vi "Add autonmous program.vi"(10 "Programs in":string[](array[string]), 11 "Program Name in":string[](array[string])) -> (2 "Programs out":string[](array[string]), 3 "Program Name out":string[](array[string]))   [LabVIEW 2013]
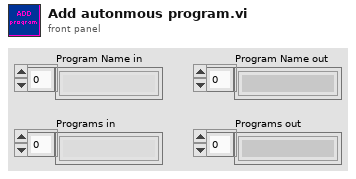
[diagram p1: front panel]
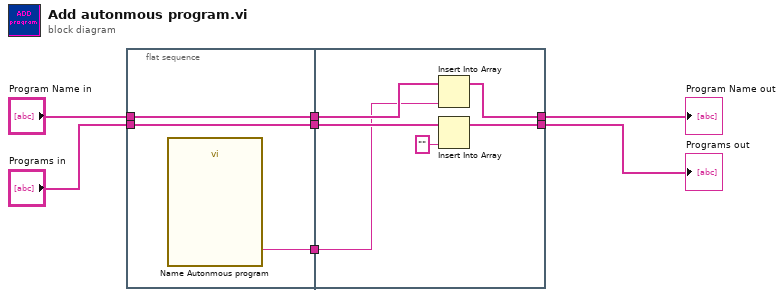
[diagram p0: block diagram]
diagram:
  n1 = flat-sequence {
    tunnel: [w10] -> w7
    tunnel: "Program Name in" -> [w10]
    tunnel: "Programs in" -> [w9]
    tunnel: [w9] -> w6
    tunnel: [w8] -> w1
    tunnel: w7 -> [w16]
    tunnel: [w15] -> w3
    tunnel: [w13] -> w5
    tunnel: w6 -> [w14]
    tunnel: w1 -> [w12]
    frame #0 {
      n2 = call "Name Autonmous program"() -> ("Autonmous Name"=w8:string)  [unwired: 17 in, 2 out]
    }
    frame #1 {
      n3 = Insert Into Array(array=w16, new element=w12) -> (w15:string[])  [unwired: 1 in]
      n4 = Insert Into Array(array=w14, new element="" ("new element/subarray")) -> (w13:string[])  [unwired: 1 in]
    }
  }
  "Programs out" <- w5
  "Program Name out" <- w3
